vi "RTS Extract TCP DBL.vi"(0 "Chamber 1 Socket":string[][](array[string]), 5 "Extract Column":i32=71, 11 "Error In":errorcluster) -> (2 "Station 1":dbl, 3 "Station 2":dbl, 4 "Station 3":dbl, 6 "Station 4":dbl, 8 "Station 5":dbl, 10 "Station 6":dbl, 13 "Station 8":dbl, 14 "Station 7":dbl, 15 "Error Out":errorcluster)   [LabVIEW 2020]
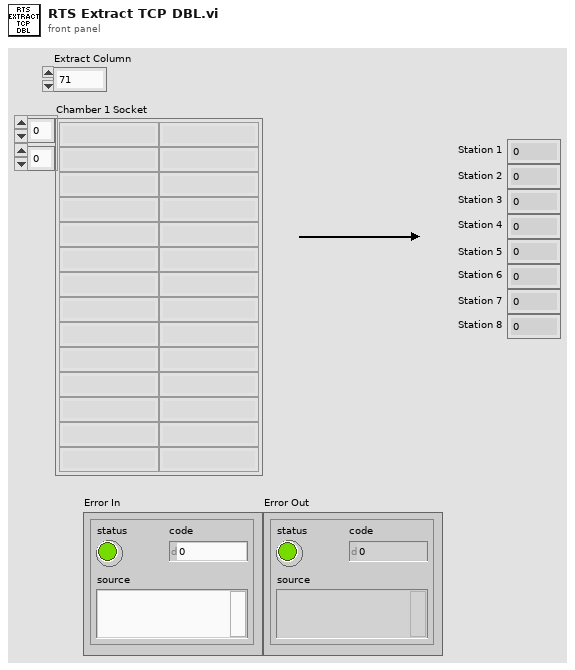
[diagram p1: front panel]
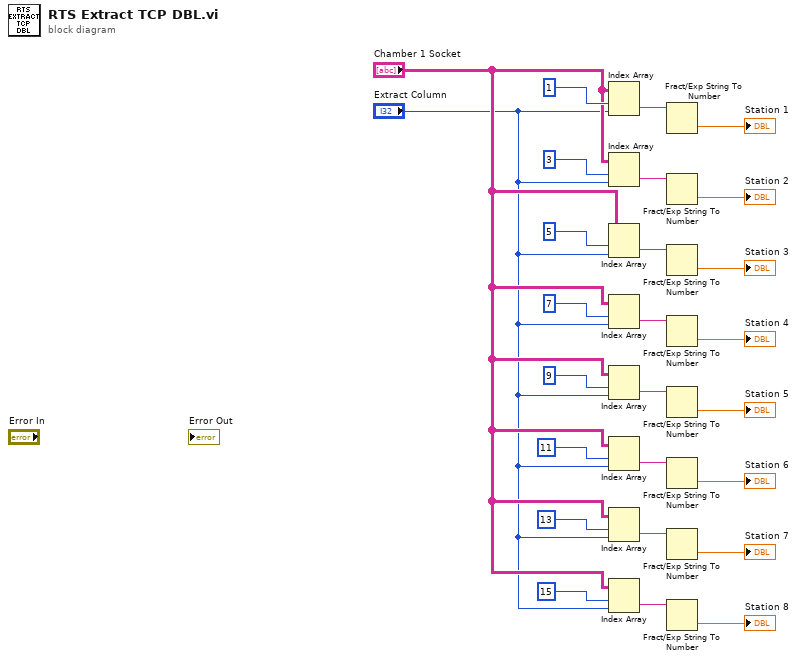
[diagram p0: block diagram]
diagram:
  n1 = Index Array(array="Chamber 1 Socket", index (row)=1, index (col)="Extract Column") -> (element=w25:string)
  n2 = Index Array(array="Chamber 1 Socket", index (row)=3, index (col)="Extract Column") -> (element=w16:string)
  n3 = Index Array(array="Chamber 1 Socket", index (row)=5, index (col)="Extract Column") -> (element=w15:string)
  n4 = Index Array(array="Chamber 1 Socket", index (row)=7, index (col)="Extract Column") -> (element=w14:string)
  n5 = Index Array(array="Chamber 1 Socket", index (row)=9, index (col)="Extract Column") -> (element=w13:string)
  n6 = Index Array(array="Chamber 1 Socket", index (row)=11, index (col)="Extract Column") -> (element=w12:string)
  n7 = Index Array(array="Chamber 1 Socket", index (row)=13, index (col)="Extract Column") -> (element=w11:string)
  n8 = Index Array(array="Chamber 1 Socket", index (row)=15, index (col)="Extract Column") -> (element=w10:string)
  n9 = Fract/Exp String To Number(string=w25) -> (number=→"Station 1":dbl)  [unwired: 3 in, 1 out]
  n10 = Fract/Exp String To Number(string=w16) -> (number=→"Station 2":dbl)  [unwired: 3 in, 1 out]
  n11 = Fract/Exp String To Number(string=w15) -> (number=→"Station 3":dbl)  [unwired: 3 in, 1 out]
  n12 = Fract/Exp String To Number(string=w14) -> (number=→"Station 4":dbl)  [unwired: 3 in, 1 out]
  n13 = Fract/Exp String To Number(string=w13) -> (number=→"Station 5":dbl)  [unwired: 3 in, 1 out]
  n14 = Fract/Exp String To Number(string=w12) -> (number=→"Station 6":dbl)  [unwired: 3 in, 1 out]
  n15 = Fract/Exp String To Number(string=w11) -> (number=→"Station 7":dbl)  [unwired: 3 in, 1 out]
  n16 = Fract/Exp String To Number(string=w10) -> (number=→"Station 8":dbl)  [unwired: 3 in, 1 out]
